vi "Drive-by-Wire passthrough.vi"(11 "stop":bool) -> ()   [LabVIEW 2014]
uses:
  <vilib>/rvi/interface/nirviOpenFPGA/nirviOpenFPGA.xnode
  <vilib>/rvi/interface/nirviReadWriteControl/nirviReadWriteControl.xnode
  <vilib>/rvi/interface/Simulation/niFpgaSimulationCallBeginRW.vi
  <vilib>/rvi/errors/niLvFpgaAdjustHostInterfaceError.vi
  <vilib>/rvi/interface/nirviCloseFPGA/nirviCloseFPGA.xnode
  <vilib>/Utility/error.llb/Error Cluster From Error Code.vi
  FPGA Bitfiles/FormulaElectric2_FPGATarget_FPGA_KFopRbsiCjk.lvbitx
  FPGA/Sensor Library/FPGA.vi
  <vilib>/FPGAPlugInAG/sbRIO-9626/niLvFpga_Open_sbRIO-9626.vi
  <vilib>/rvi/interface/common/dynamic/niFpgaDynamicAddResources.vi
  NiFpgaLv.dll
  <vilib>/FPGAPlugInAG/Dynamic/niLvFpga_Close_Dynamic.vi
panel:
  in  "cRIO Shutdown 2":bool=TRUE
  in  "cRIO Shutdown 1":bool=TRUE
  out "Throttle 2 (%)":fxp<+/-,45,19>
  out "Throttle 1 (%)":fxp<+/-,45,19>
  in  "Throttle 2 Max":fxp<+,16,4>=2.300048828125
  in  "Throttle 2 Min":fxp<+,16,4>=0.5
  out "Throttle 2 (V)":fxp<+/-,26,5>
  out "Throttle1 (V)":fxp<+/-,26,5>=4.955944061279297
  in  "Throttle1 Max":fxp<+,16,4>=2.300048828125
  in  "Throttle1 Min":fxp<+,16,4>=0.5
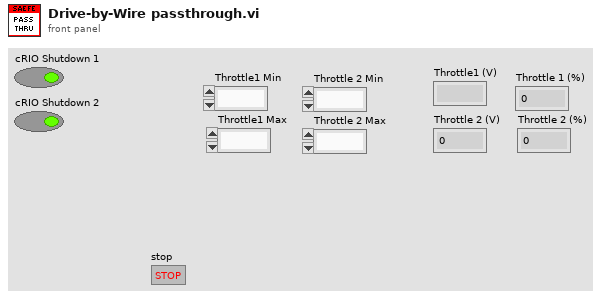
[diagram p1: front panel]
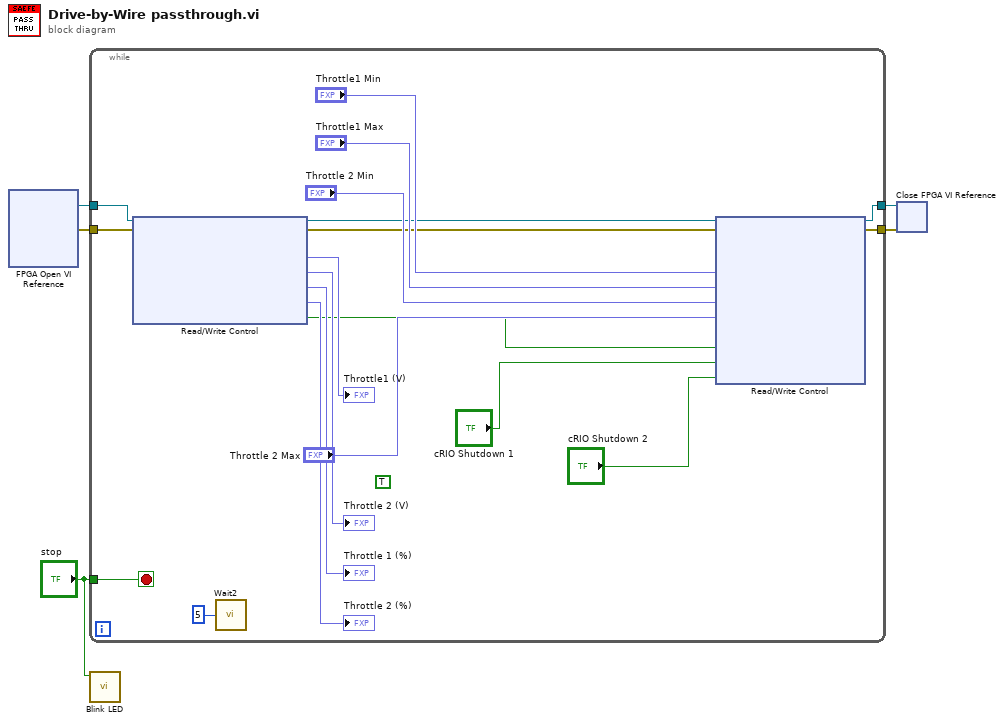
[diagram p0: block diagram]
diagram:
  n1 = xnode "FPGA Open VI Reference"() -> ("FPGA VI Reference Out"=w5:refnum<k20>, "error out"=w3:errorcluster)  [unwired: 2 in]
  n2 = while {
    tunnel: w5 -> [w24]
    tunnel: [w23] -> w4
    tunnel: w3 -> [w22]
    tunnel: [w21] -> w2
    tunnel: "stop" -> [w17]
    stop <- w17 stop-if-true
    (unwired) TRUE ("Override Throttle Checks")
    n3 = xnode "Read/Write Control"("FPGA VI Reference In"=w24, "error in"=w22) -> ("FPGA VI Reference Out"=w10:refnum<k20>, "error out"=w9:errorcluster, "Throttle 1 (V)"=→"Throttle1 (V)":fxp<+/-,24,5>, "Throttle 2 (V)"=→"Throttle 2 (V)":fxp<+/-,24,5>, "Throttle 1 (%)"=→"Throttle 1 (%)":fxp<+/-,27,18>, "Throttle 2 (%)"=→"Throttle 2 (%)":fxp<+/-,27,18>, "Motor Controller Dash Switch"=w8:bool)  [unwired: 1 out]
    n4 = call "Wait2"("Count(mSec)"=u32 5) -> ()  [unwired: 1 out]
    n5 = xnode "Read/Write Control"("FPGA VI Reference In"=w10, "error in"=w9, "Throttle 1 Min"="Throttle1 Min", "Throttle 1 Max"="Throttle1 Max", "Throttle 2 Min"="Throttle 2 Min", "Throttle 2 Max"="Throttle 2 Max", "Motor Controller Power"=w8, "cRIO Shutdown 1"="cRIO Shutdown 1", "cRIO Shutdown 2"="cRIO Shutdown 2") -> ("FPGA VI Reference Out"=w23:refnum<k20>, "error out"=w21:errorcluster)  [unwired: 3 in]
  }
  n6 = call "Blink LED.vi"("stop"="stop") -> ()  [unwired: 11 in]
  n7 = xnode "Close FPGA VI Reference"("FPGA VI Reference In"=w4, "error in"=w2) -> ()  [unwired: 1 out]
